vi "Log To Spreadsheet File.vi"(8 "error in (no error)":errorcluster, 9 "spreadsheet string":string, 10 "append to file? (new file:F)":bool, 11 "file path (dialog if empty)":path) -> (0 "error out":errorcluster, 3 "new file path (Not A Path if cancelled)":path)   [LabVIEW 2015]
doc: "Converts a 2D or 1D array of strings, signed integers, or double-precision numbers to a text string and writes the string to a new byte stream file or appends the string to an existing file. \n\nWire data to the <B>2D data</B> input or <B>1D data</B> input to determine the polymorphic instance to use or manually select the instance."
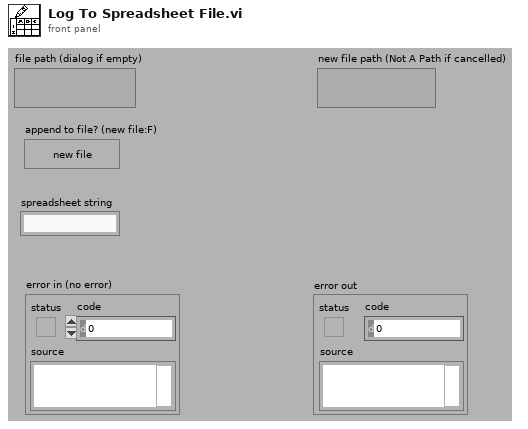
[diagram p1: front panel]
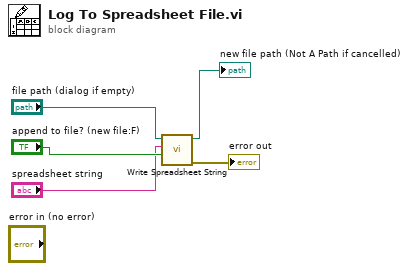
[diagram p0: block diagram]
diagram:
  n1 = call <vilib>:"Write Spreadsheet String.vi"("append to file? (new file:F)"="append to file? (new file:F)", "spreadsheet string"="spreadsheet string", "file path (dialog if empty)"="file path (dialog if empty)") -> ("error out"=→"error out":errorcluster, "path"=→"new file path (Not A Path if cancelled)":path)  [unwired: 7 in]
